vi "Global.exit.vi"() -> ()   [LabVIEW 2019]
panel:
  in  "Exit":bool
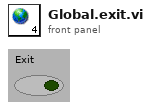
[diagram p1: front panel]
diagram:
